vi "GryoMoveForward.vi"() -> ()   [LabVIEW 2016, in "LEGO-PMR.lvrbt"]
uses:
  LEGO-PMR.lvrbt
  <vilib>/NXT/Block Support/NXT_InputPort.ctl
  <vilib>/NXT/Block Support/NXT_OutputPort.ctl
  <vilib>/NXT/Dual Mode Library/Sensors/EV3_Gyro_Reset.vi
  <vilib>/NXT/NXTIO Xnodes/NXTIONodeSubVIs/LEGOResetMotors.vi
  <vilib>/NXT/Dual Mode Library/Waits/Wait_Num(msec).vi
  <vilib>/NXT/NXTIO Xnodes/NXTIONodeSubVIs/LEGOMotorStatus.vi
  <vilib>/NXT/Dual Mode Library/Sensors/EV3_Gyro_Angle.vi
  <vilib>/NXT/NXTIO Xnodes/NXTIONodeSubVIs/NXTMoveMotors.vi
  <vilib>/NXT/NXTIO Xnodes/AddressXNode/NXTIOAddress.xnode
  <vilib>/NXT/NXTIO Xnodes/NXTIOXNode/NXTIO.xnode
  <vilib>/NXT/Subs/LVHSConnector.ctl
  <vilib>/NXT/LegoClasses/BrickReference/BrickReference.lvclass
panel:
  out "Gain":dbl
  out "Read Angle":dbl
  in  "Speed":dbl
  in  "Angle":dbl
  in  "Distance":dbl
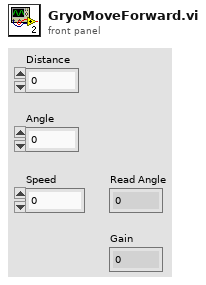
[diagram p1: front panel]
types:
  T1 = typedef "NXT_InputPort.ctl" = u32
  T2 = typedef "LVHSConnector.ctl" = refnum<class "BrickReference.lvclass">
  T3 = typedef "NXT_OutputPort.ctl" = u8
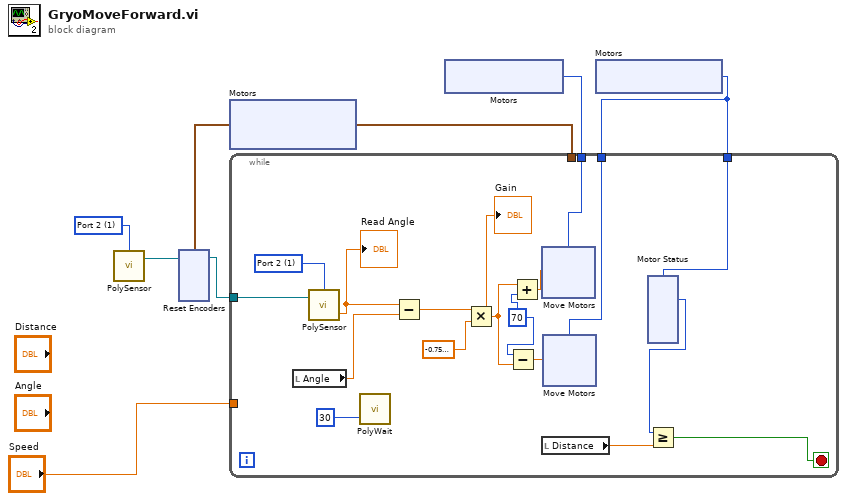
[diagram p0: block diagram]
diagram:
  w6 = T1 1 items=["Port 1", "Port 2", "Port 3", "Port 4"] ("Port (Port 1)")
  n1 = call-poly <vilib>:"PolySensor.vi"("Port (Port 1)"=w6) -> ("NXT/EV3"=w7:T2)  [unwired: 3 in]
  n2 = xnode "Motors"() -> ("Motor"=w5:cluster{"Port":T3, "Port":T3})
  n3 = xnode "Reset Encoders"("Motors"=w5, "NXT/EV3"=w7) -> ("NXT/EV3"=w4:T2)
  n4 = xnode "Motors"() -> ("Motor"=w2:T3)
  n5 = xnode "Motors"() -> ("Motor"=w1:T3)
  n6 = while {
    tunnel: w5 -> [_]
    tunnel: w4 -> [w20]
    tunnel: "Speed" -> [_]
    tunnel: w2 -> [w16]
    tunnel: w1 -> [w15]
    tunnel: w1 -> [w14]
    stop <- w18 stop-if-true
    w11 = 70
    w24 = T1 1 items=["Port 1", "Port 2", "Port 3", "Port 4"] ("Port (Port 1)")
    n7 = local read "Angle"() -> (w23:dbl)
    n8 = call-poly <vilib>:"PolySensor.vi"("NXT/EV3"=w20, "Port (Port 1)"=w24) -> ("Degrees"=w17:sgl)  [unwired: 1 in, 1 out]
    "Read Angle" <- w17
    n9 = call-poly <vilib>:"PolyWait.vi"("Time (100 msec)"=u32 30 ("Time (1 sec)")) -> ()  [unwired: 3 in, 1 out]
    n10 = Subtract(x=w17, y=w23) -> (x-y=w21:dbl)
    n11 = Multiply(x=w21, y=-0.7500000000000002) -> (x*y=w10:dbl)
    "Gain" <- w10
    n12 = Subtract(x=w11, y=w10) -> (x-y=w9:dbl)
    n13 = Add(x=w10, y=w11) -> (x+y=w8:dbl)
    n14 = xnode "Move Motors"("Power/Speed 1"=w8, "Motors"=w16) -> ()  [unwired: 1 in, 1 out]
    n15 = local read "Distance"() -> (w19:dbl)
    n16 = xnode "Move Motors"("Power/Speed 1"=w9, "Motors"=w15) -> ()  [unwired: 1 in, 1 out]
    n17 = xnode "Motor Status"("Motors"=w14) -> ("Position 1"=w13:i32)  [unwired: 1 in, 2 out]
    n18 = Greater Or Equal?(x=w13, y=w19) -> (x >= y?=w18:bool)
  }
